vi "Configure Sine Out.vi"(7 "Sine Out DC Level Mode (0: Common)":i32(ring) items=["Common", "Difference"], 8 "error in (no error)":errorcluster, 9 "Sine Out DC Level to Voltage (0 V)":dbl format="%#_6f", 10 "Sine Out Amplitude to Voltage (0 V)":dbl, 11 "VISA resource name":refnum<visa-resource-name>) -> (3 "VISA resource name out":refnum<visa-resource-name>)   [LabVIEW 2020, in "Stanford Research SR865.lvlib"]
doc: "Configures the sine output reference source."
uses:
  Stanford Research SR865.lvlib
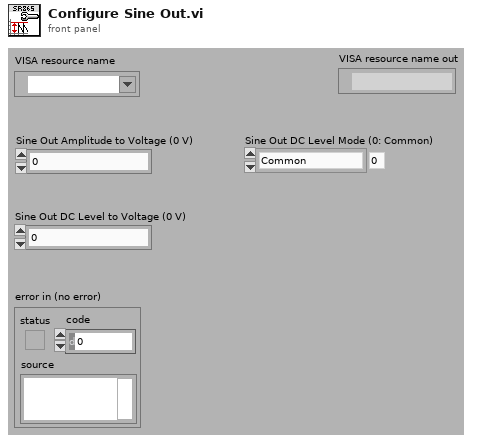
[diagram p1: front panel]
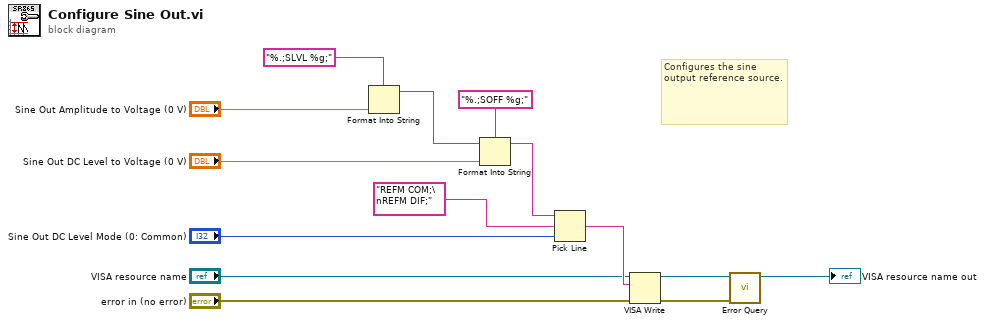
[diagram p0: block diagram]
diagram:
  # "Configures the sine output reference source."
  n1 = Format Into String(format string="%.;SLVL %g;", "Sine Out Amplitude to Voltage (0 V)") -> (resulting string=w13:string)  [unwired: 2 in, 1 out]
  n2 = Format Into String(format string="%.;SOFF %g;", initial string=w13, "Sine Out DC Level to Voltage (0 V)") -> (resulting string=w2:string)  [unwired: 1 in, 1 out]
  n3 = Pick Line(string ("")=w2, multi-line string="REFM COM;\nREFM DIF;", line index="Sine Out DC Level Mode (0: Common)") -> (output string=w8:string)
  n4 = VISA Write(VISA resource name="VISA resource name", write buffer=w8, error in (no error)="error in (no error)") -> (VISA resource name out=w5:refnum<visa-resource-name>, error out=w4:errorcluster)  [unwired: 1 out]
  n5 = call "Error Query.vi"("error in (no error)"=w4, "VISA resource name"=w5) -> ("VISA resource name out"=→"VISA resource name out":refnum<visa-resource-name>)  [unwired: 7 in, 2 out]
